vi "Initialise.vi"(8 "error in (no error)":errorcluster, 10 "Message in":refnum<class "InitialiseMessage.lvclass">, 11 "ImageStack in":refnum<class "Invivo_ImageStack.lvclass">) -> (0 "error out":errorcluster, 3 "ImageStack out":refnum<class "Invivo_ImageStack.lvclass">)   [LabVIEW 2012, in "Invivo_ImageStack.lvclass"]
doc: "This method is called when an initialise message is received. It mainly initialises the RabbitMQ connectivity. \n\nOverride this method when your component needs special initialisation (e.g. of software or hardware resources). In that case, don't forget to call the parent for proper implementation. If your component owns subcomponents, they count as resources, so you have to initialise them by calling their own initialise functions"
uses:
  Invivo_ImageStack.lvclass
  <vilib>/Distrio/Murmex/InitialiseMessage/InitialiseMessage.lvclass
  <vilib>/Distrio/Murmex/Murmex/Murmex.lvclass
  <vilib>/Distrio/Murmex/Murmex/update_cluster.ctl
  <vilib>/Distrio/Murmex/GenericMessage/GenericMessage.lvclass
  Invivo_ImageStack.lvclass/Invivo_ImageStack.ctl
  <vilib>/Distrio/Murmex/Message/Add or replace parameter.vi
panel:
  # "This method is called when the INTIALISE\ntrigger is sent. \n\nOverride this method when your component needs to\nrespond to this trigger. \n\nCall parent for proper implementation"
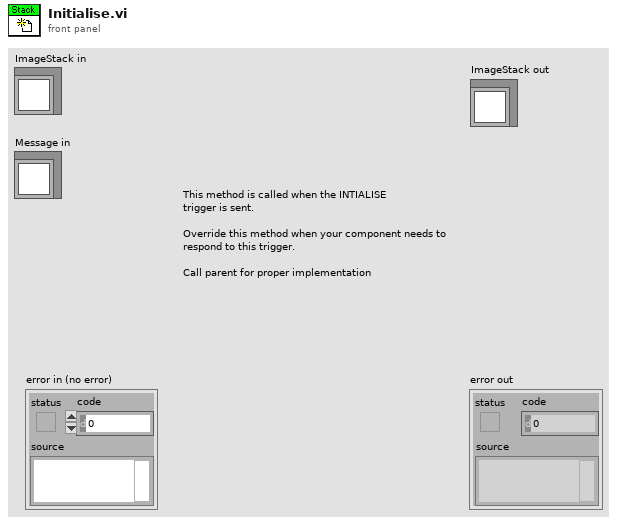
[diagram p1: front panel]
types:
  T1 = typedef "Murmex.lvlib/Murmex.lvclass/update_cluster.ctl" = cluster{"target ID":string, "key chains":string[], "values":variant[]}
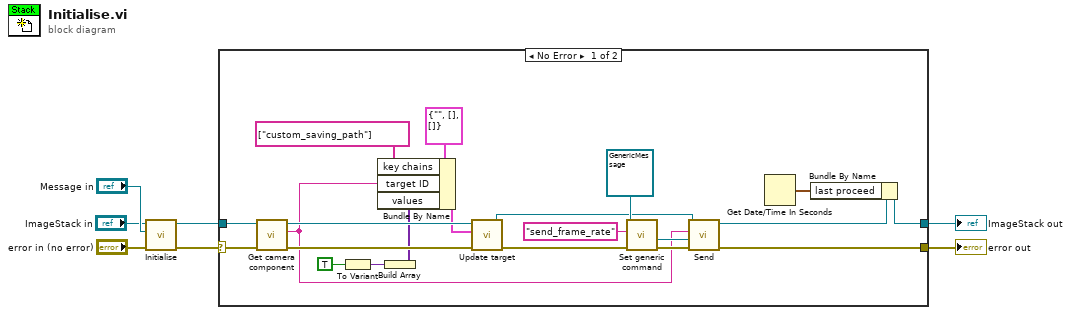
[diagram p0: block diagram]
diagram:
  n1 = call-parent "Initialise.vi"("error in (no error)"="error in (no error)", "Message in"="Message in", "Murmex in"="ImageStack in") -> ("error out"=w4:errorcluster, "Murmex out"=w1:refnum<class "Invivo_ImageStack.lvclass">)  [unwired: 7 in]
  n2 = case shown="No Error" w4 {
    selector: w4 -> [w28 w30]
    tunnel: [w14 w30] -> w3
    tunnel: [w9 w29] -> w2
    tunnel: w1 -> [w27 w29]
    frame No Error {
      n3 = call-dynamic "Get camera component.vi"("error in (no error)"=w28, "ImageStack in"=w27) -> ("error out"=w26:errorcluster, "Camera component name"=w12:string, "ImageStack out"=w25:refnum<class "Invivo_ImageStack.lvclass">)  [unwired: 7 in]
      n4 = To Variant(anything=TRUE) -> (Variant=w20:variant)
      n5 = Build Array(w20) -> (w19:variant[])
      n6 = Bundle By Name(cluster=T1 {"target ID"="", "key chains"=[], "values"=[]} ("update cluster"), "key chains"=string[] ["custom_saving_path"], "target ID"=w12, "values"=w19) -> (w23:T1)
      n7 = call <vilib>:"Update target.vi"("error in (no error)"=w26, "update cluster"=w23, "MurmexBase in"=w25) -> ("error out"=w16:errorcluster, "MurmexBase out"=w11:refnum<class "Invivo_ImageStack.lvclass">)  [unwired: 7 in]
      n8 = call <vilib>:"Set generic command.vi"("error in (no error)"=w16, "generic command"="send_frame_rate", "GenericMessage in"=refnum<class "GenericMessage.lvclass"> refnum ("Distrio Murmex 1.1:GenericMessage")) -> ("error out"=w15:errorcluster, "GenericMessage out"=w13:refnum<class "GenericMessage.lvclass">)  [unwired: 7 in]
      n9 = call <vilib>:"Send.vi"("error in (no error)"=w15, "Message"=w13, "recipient"=w12, "Murmex in"=w11) -> ("error out"=w14:errorcluster, "Murmex out"=w10:refnum<class "Invivo_ImageStack.lvclass">)  [unwired: 6 in]
      n10 = Get Date/Time In Seconds() -> (seconds since 1Jan1904=w8:timestamp)
      n11 = Bundle By Name(cluster=w10, "last proceed"=w8) -> (w9:refnum<class "Invivo_ImageStack.lvclass">)
    }
    frame Error {
    }
  }
  "error out" <- w3
  "ImageStack out" <- w2
